vi "printLog.vi"(8 "error in (no error)":errorcluster, 11 "Log in":refnum<class "Log.lvclass">) -> (0 "error out":errorcluster, 2 "String":string, 3 "Log out":refnum<class "Log.lvclass">)   [LabVIEW 2009, in "Tools.lvlib" / "xml.lvlib" / "Log.lvclass"]
uses:
  Log.lvclass
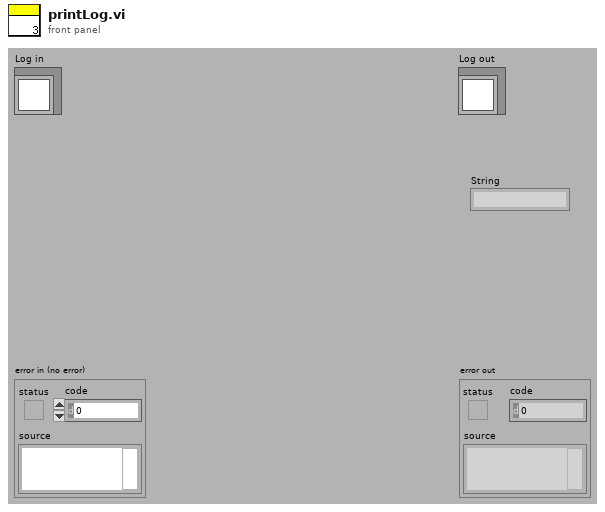
[diagram p1: front panel]
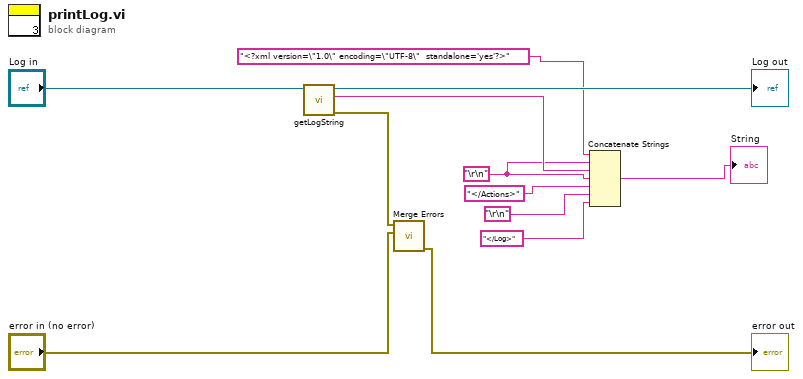
[diagram p0: block diagram]
diagram:
  w1 = "\r\n"
  n1 = call-dynamic "getLogString.vi"("Log.lvclass in"="Log in") -> ("error out"=w10:errorcluster, "logString"=w7:string, "Log.lvclass out"=→"Log out":refnum<class "Log.lvclass">)  [unwired: 8 in]
  n2 = call <vilib>:"Merge Errors.vi"("error in 2 (no error)"="error in (no error)", "error in 1 (no error)"=w10) -> ("error out"=→"error out":errorcluster)  [unwired: 5 in]
  n3 = Concatenate Strings("<?xml version=\"1.0\" encoding=\"UTF-8\"  standalone='yes'?>", w1, w7, w1, "</Actions>", "\r\n", "</Log>") -> (→"String":string)
